vi "Execute.vi"(8 "error in (no error)":errorcluster, 9 "Targets":T1[](array[typedef]), 11 "Project Path":path) -> (0 "error out":errorcluster)   [LabVIEW 2015, in "Project.lvclass"]
uses:
  Project.lvclass
  FPGA Settings.ctl
  Module/Module/Module Settings.ctl
  Signal/Signal/Signal Settings.ctl
  Read Folder Ref.vi
  VI/VI/VI.lvclass
  Signal/Signal/Signal.lvclass
  Module/Module/Module.lvclass
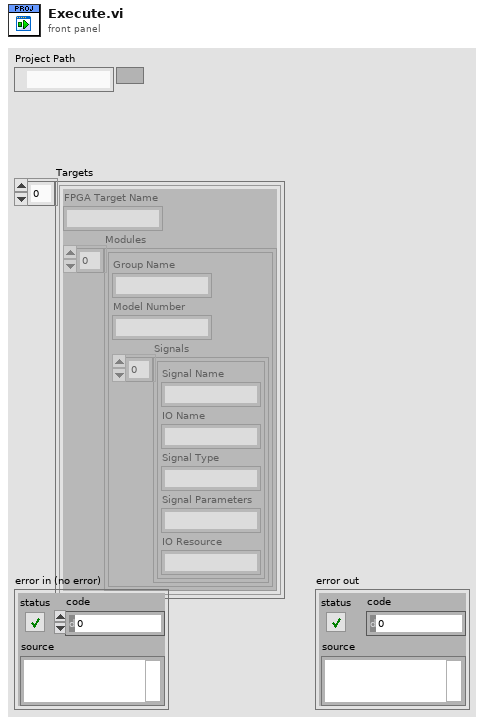
[diagram p1: front panel]
types:
  T1 = typedef "Project.lvclass/FPGA Settings.ctl" = cluster{"FPGA Target Name":string, "Modules":T2[]}
  T2 = typedef "Module.lvclass/Module Settings.ctl" = cluster{"Group Name":string, "Model Number":string, "Signals":T3[]}
  T3 = typedef "Signal.lvclass/Signal Settings.ctl" = cluster{"Signal Name":string, "IO Name":string, "Signal Type":string, "Signal Parameters":string, "IO Resource":string}
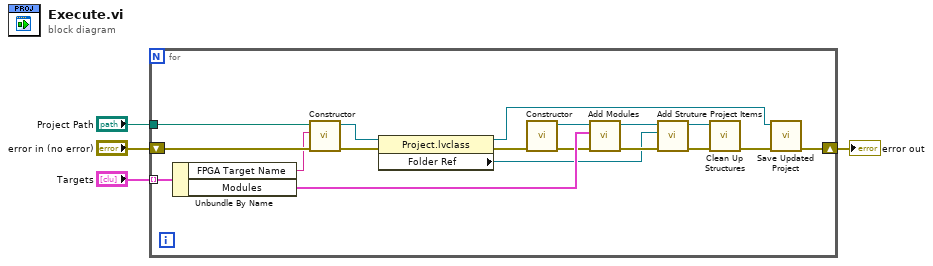
[diagram p0: block diagram]
diagram:
  n1 = for {
    tunnel: "Project Path" -> [w22]
    shift-right: [w9] -> w2
    shift-left: "error in (no error)" -> [w17]
    tunnel: "Targets" -> [w16] mode=indexing
    n2 = Unbundle By Name(w16) -> ("FPGA Target Name"=w15:string, "Modules"=w14:T2[])
    n3 = call "Constructor.vi"("error in (no error)"=w17, "FPGA Target Name"=w15, "Project Path"=w22) -> ("error out"=w20:errorcluster, "Project out"=w21:refnum<class "Project.lvclass">)  [unwired: 7 in]
    n4 = property class="Project.lvclass"(reference=w21, error in=w20) -> (reference out=w18:refnum<class "Project.lvclass">, error out=w19:errorcluster, "Folder Ref"=w5:refnum<vi>)
    n5 = call "Constructor.vi"("error in (no error)"=w19) -> ("error out"=w11:errorcluster, "Block Diagram"=w10:refnum<class "VI.lvclass">)  [unwired: 9 in]
    n6 = call "Add Modules.vi"("error in (no error)"=w11, "Modules"=w14, "Block Diagram in"=w10) -> ("error out"=w12:errorcluster, "Block Diagram out"=w13:refnum<class "VI.lvclass">)  [unwired: 7 in]
    n7 = call "Add Struture Project Items.vi"("error in (no error)"=w12, "Folder Location Ref"=w5, "Block Diagram in"=w13) -> ("error out"=w8:errorcluster, "Block Diagram out"=w6:refnum<class "VI.lvclass">)  [unwired: 7 in]
    n8 = call "Clean Up Structures.vi"("error in (no error)"=w8, "Block Diagram in"=w6) -> ("error out"=w7:errorcluster)  [unwired: 8 in, 1 out]
    n9 = call-dynamic "Save Updated Project.vi"("error in (no error)"=w7, "Project in"=w18) -> ("error out"=w9:errorcluster)  [unwired: 8 in, 1 out]
  }
  "error out" <- w2
